vi "Load.vi"(0 "Robot Event Local Log in":refnum<class "Robot Event Local Log.lvclass">, 1 "Event Parameters":T1[](array[typedef]), 5 "error in (no error)":errorcluster) -> (14 "Robot Event Local Log out":refnum<class "Robot Event Local Log.lvclass">, 19 "error out":errorcluster)   [LabVIEW 2019, in "Robot Event Local Log.lvclass"]
uses:
  Robot Event Local Log.lvclass
  Robot Event/Event Parameters.ctl
  Robot Event Local Log.lvclass/Robot Event Local Log.ctl
  Robot Event/Robot Event.lvclass
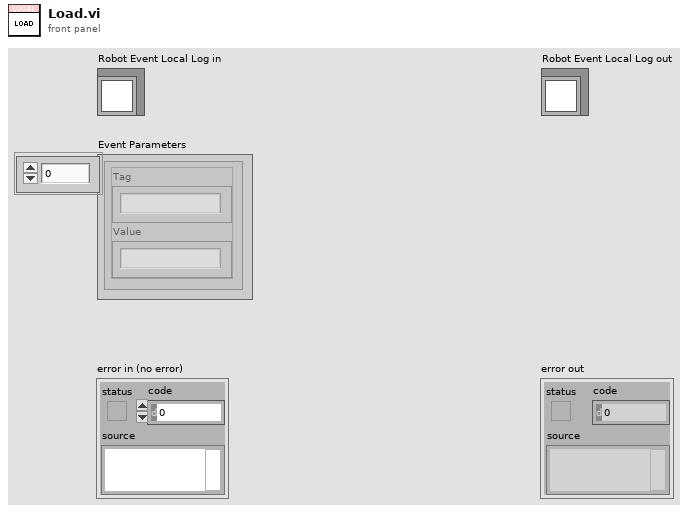
[diagram p1: front panel]
types:
  T1 = typedef "Robot Event.lvclass/Event Parameters.ctl" = cluster{"Tag":string, "Value":string}
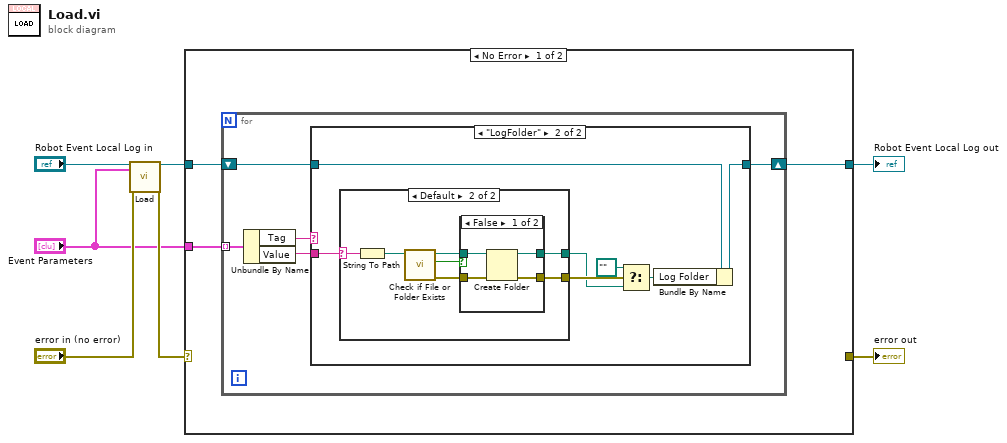
[diagram p0: block diagram]
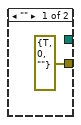
[diagram p3: hidden frame]
diagram:
  n1 = call-parent "Load.vi"("Robot Event in"="Robot Event Local Log in", "Event Parameters"="Event Parameters", "error in (no error)"="error in (no error)") -> ("Robot Event out"=w4:refnum<class "Robot Event Local Log.lvclass">, "error out"=w3:errorcluster)  [unwired: 15 in]
  n2 = case shown="No Error" w3 {
    selector: w3 -> [_ w39]
    tunnel: [_ w39] -> w7
    tunnel: [w9 w38] -> w6
    tunnel: w4 -> [w10 w38]
    tunnel: "Event Parameters" -> [w8 _]
    frame No Error {
      n3 = for {
        shift-right: [w14] -> w9
        shift-left: w10 -> [w15]
        tunnel: w8 -> [w13] mode=indexing
        n4 = Unbundle By Name(w13) -> ("Tag"=w12:string, "Value"=w11:string)
        n5 = case shown="\"LogFolder\"" w12 {
          tunnel: w15 -> [w16 w23]
          tunnel: [w16 w22] -> w14
          tunnel: w11 -> [_ w21]
          frame Default {
          }
          frame "LogFolder" {
            n6 = case shown="Default" w21 {
              selector: w21 -> [_ w26]
              tunnel: [_ w27] -> w19
              tunnel: [errorcluster {"status"=TRUE, "code"=0, "source"=""} ("error out") w25] -> w20
              frame "" {
              }
              frame Default {
                n7 = String To Path(string=w26) -> (path=w28:path)
                n8 = call <vilib>:"Check if File or Folder Exists.vi"("path"=w28) -> ("error out"=w29:errorcluster, "file or folder exists?"=w31:bool, "dup path"=w30:path)  [unwired: 8 in]
                n9 = case shown="False" w31 {
                  tunnel: w30 -> [w34 w36]
                  tunnel: w29 -> [w35 w37]
                  tunnel: [w33 w37] -> w25
                  tunnel: [w32 w36] -> w27
                  frame False {
                    n10 = Create Folder(path (use dialog)=w34, error in=w35) -> (created path=w32:path, error out=w33:errorcluster)  [unwired: 1 in, 1 out]
                  }
                  frame True {
                  }
                }
              }
            }
            n11 = Select(t=path "", s=w20, f=w19) -> (s? t:f=w18:path)
            n12 = Bundle By Name(cluster=w23, "Log Folder"=w18) -> (w22:refnum<class "Robot Event Local Log.lvclass">)
          }
        }
      }
    }
    frame Error {
    }
  }
  "error out" <- w7
  "Robot Event Local Log out" <- w6
